vi "sendValue.vi"(8 "error in (no error)":errorcluster, 10 "data":variant, 11 "stopAzimuth in":refnum<class "stopAzimuth.lvclass">) -> (0 "error out":errorcluster, 2 "function return":i32, 3 "stopAzimuth out":refnum<class "stopAzimuth.lvclass">)   [LabVIEW 2016, in "SALLV_AtDome_Messaging.lvlib" / "stopAzimuth.lvclass"]
uses:
  stopAzimuth.lvclass
  ts_sallv_AtDome/DataTypes/command_stopAzimuth.ctl
  ts_sallv_AtDome/SALLV_AtDome.lvlib
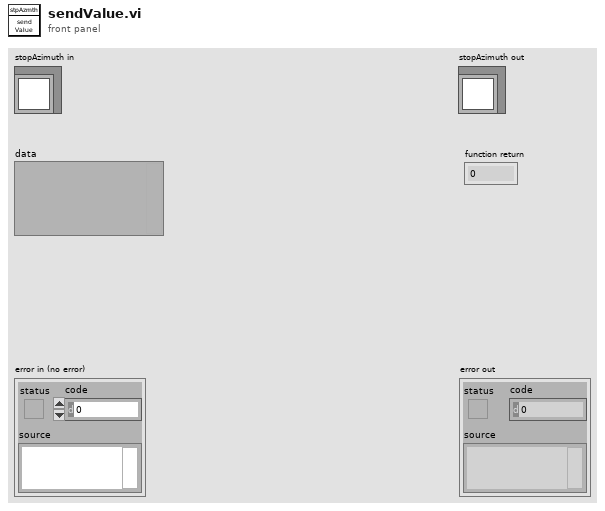
[diagram p1: front panel]
types:
  T1 = typedef "SALLV_AtDome.lvlib/command_stopAzimuth.ctl" = cluster{"value":bool}
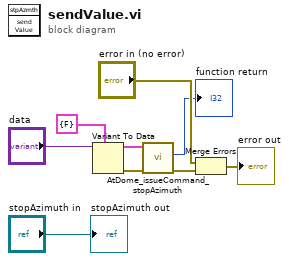
[diagram p0: block diagram]
diagram:
  n1 = Variant To Data(type=T1 {"value"=FALSE} ("data"), Variant="data") -> (data=w4:T1, error out=w5:errorcluster)  [unwired: 1 in]
  n2 = call "AtDome_issueCommand_stopAzimuth.vi"("error in (no error)"=w5, "command_stopAzimuth_Ctl"=w4) -> ("error out"=w2:errorcluster, "function return"=→"function return":i32)  [unwired: 7 in, 1 out]
  n3 = Merge Errors("error in (no error)", w2) -> (→"error out":errorcluster)
  "stopAzimuth out" <- "stopAzimuth in"
